vi "generateSignedStrings.vi"(6 "timeout (10000)":i32=10000, 8 "error in (no error)":errorcluster, 11 "Parameters":T2={"params"={"apiKey"="", "n"=0, "length"=0, "characters"="", "replacement"=TRUE}, "id"=0.0}) -> (0 "error out":errorcluster, 3 "Response":T1={"result"={"random"={"method"="", "hashedApiKey"="", "n"=0, "length"=0, "characters"="", "replacement"=TRUE, "data"=[], "completionTime"="", "serialNumber"=0}, "signature"="", "bitsUsed"=0, "bitsLeft"=0, "requestsLeft"=0, "advisoryDelay"=0}, "id"=0.0}, 4 "error data":string[](array[string]))   [LabVIEW 2017, in "Random JSON API.lvlib"]
uses:
  Random JSON API.lvlib
  Type Defs/generateStringsRequest.ctl
  Type Defs/generateSignedStringsResponse.ctl
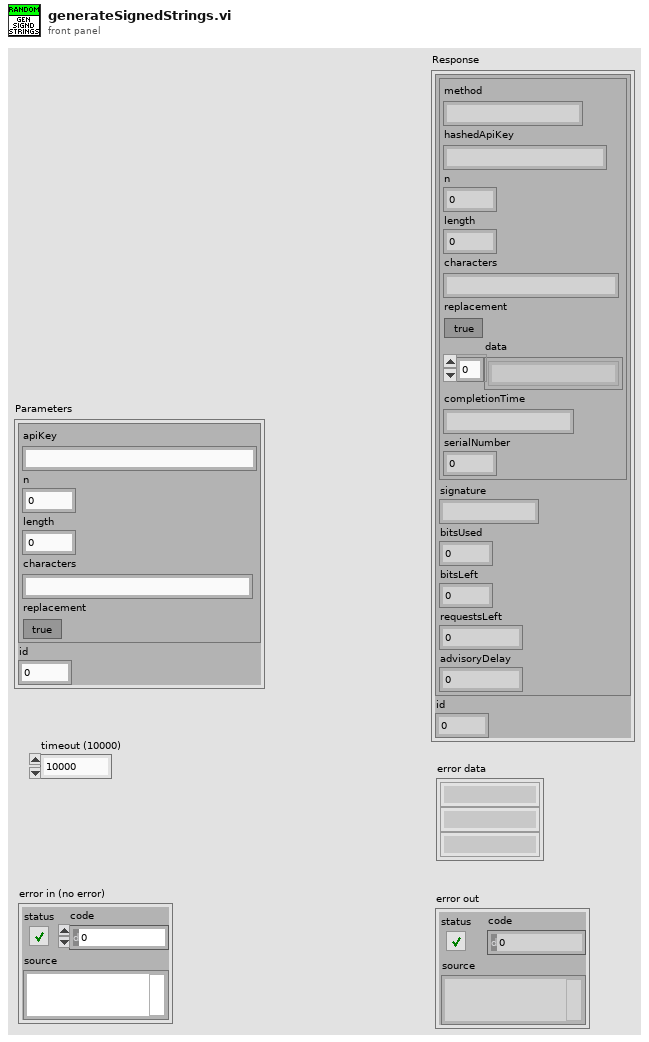
[diagram p1: front panel]
types:
  T1 = typedef "Random JSON API.lvlib/generateSignedStringsResponse.ctl" = cluster{"result":cluster{"random":cluster{"method":string, "hashedApiKey":string, "n":i32, "length":i32, "characters":string, "replacement":bool, "data":string[], "completionTime":string, "serialNumber":i32}, "signature":string, "bitsUsed":i32, "bitsLeft":i32, "requestsLeft":i32, "advisoryDelay":i32}, "id":dbl}
  T2 = typedef "Random JSON API.lvlib/generateStringsRequest.ctl" = cluster{"params":cluster{"apiKey":string, "n":i32, "length":i32, "characters":string, "replacement":bool}, "id":dbl}
  T3 = cluster{"apiKey":string, "n":i32, "length":i32, "characters":string, "replacement":bool}
  T4 = cluster{"jsonrpc":string, "method":string, "params":cluster{"apiKey":string, "n":i32, "length":i32, "characters":string, "replacement":bool}, "id":dbl}
  T5 = cluster{"result cluster":cluster{"completionTime":string, "bitsUsed":i32, "bitsLeft":i32, "requestsLeft":i32, "advisoryDelay":i32}, "method":string, "hashedApiKey":string, "n":i32, "serialNumber":i32, "signature":string}
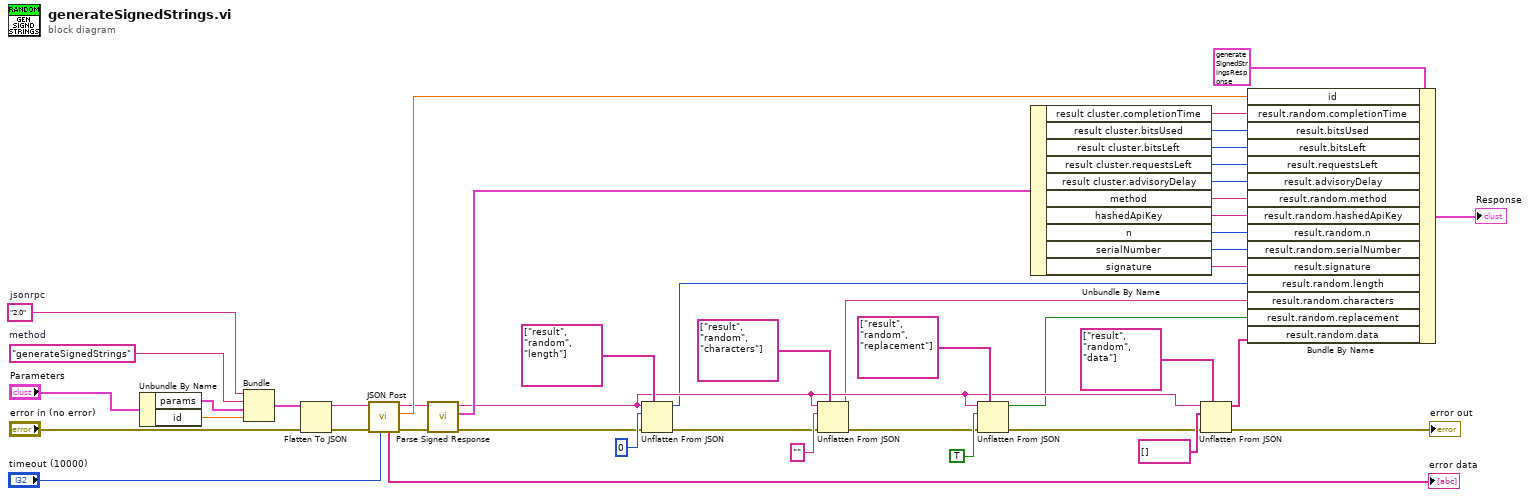
[diagram p0: block diagram]
diagram:
  w38 = "2.0"  # jsonrpc
  w37 = "generateSignedStrings"  # method
  n1 = Unbundle By Name("Parameters") -> ("params"=w36:T3, "id"=w35:dbl)
  n2 = Bundle("jsonrpc"=w38, "method"=w37, "params"=w36, "id"=w35) -> (w32:T4)  [unwired: 1 in]
  n3 = Flatten To JSON(anything=w32, error in (no error)="error in (no error)") -> (JSON string=w33:string, 11:w34:errorcluster)  [unwired: 1 in]
  n4 = call "JSON Post.vi"("timeout (10000)"="timeout (10000)", "error in (no error)"=w34, "Request JSON String"=w33) -> ("error out"=w44:errorcluster, "id"=w27:dbl, "Response JSON String"=w26:string, "error data"=→"error data":string[])  [unwired: 5 in]
  n5 = call "Parse Signed Response.vi"("error in (no error)"=w44, "body in"=w26) -> ("error out"=w8:errorcluster, "signed result cluster"=w28:T5, "body out"=w4:string)  [unwired: 7 in]
  n6 = Unflatten From JSON(path=string[] ["result", "random", "length"], JSON string=w4, type and defaults=0, error in (no error)=w8) -> (value=w1:i32, error out=w7:errorcluster)  [unwired: 3 in]
  n7 = Unflatten From JSON(path=string[] ["result", "random", "characters"], JSON string=w4, type and defaults="", error in (no error)=w7) -> (value=w2:string, error out=w6:errorcluster)  [unwired: 3 in]
  n8 = Unflatten From JSON(path=string[] ["result", "random", "replacement"], JSON string=w4, type and defaults=TRUE, error in (no error)=w6) -> (value=w3:bool, error out=w5:errorcluster)  [unwired: 3 in]
  n9 = Unbundle By Name(w28) -> ("result cluster.completionTime"=w43:string, "result cluster.bitsUsed"=w42:i32, "result cluster.bitsLeft"=w41:i32, "result cluster.requestsLeft"=w40:i32, "result cluster.advisoryDelay"=w39:i32, "method"=w19:string, "hashedApiKey"=w18:string, "n"=w17:i32, "serialNumber"=w16:i32, "signature"=w15:string)
  n10 = Unflatten From JSON(path=string[] ["result", "random", "data"], JSON string=w4, type and defaults=string[] [], error in (no error)=w5) -> (value=w20:string[], error out=→"error out":errorcluster)  [unwired: 3 in]
  n11 = Bundle By Name(cluster=T1 {"result"={"random"={"method"="", "hashedApiKey"="", "n"=0, "length"=0, "characters"="", "replacement"=TRUE, "data"=[], "completionTime"="", "serialNumber"=0}, "signature"="", "bitsUsed"=0, "bitsLeft"=0, "requestsLeft"=0, "advisoryDelay"=0}, "id"=0.0} ("Response"), "id"=w27, "result.random.completionTime"=w43, "result.bitsUsed"=w42, "result.bitsLeft"=w41, "result.requestsLeft"=w40, "result.advisoryDelay"=w39, "result.random.method"=w19, "result.random.hashedApiKey"=w18, "result.random.n"=w17, "result.random.serialNumber"=w16, "result.signature"=w15, "result.random.length"=w1, "result.random.characters"=w2, "result.random.replacement"=w3, "result.random.data"=w20) -> (→"Response":T1)
